vi "Finish.vi"(8 "error in (no error)":errorcluster, 11 "DriverStation in":refnum<class "DriverStation.lvclass">) -> (0 "error out":errorcluster, 3 "DriverStation out":refnum<class "DriverStation.lvclass">)   [LabVIEW 2013, in "DriverStation.lvclass"]
uses:
  DriverStation.lvclass
  System/System.lvclass
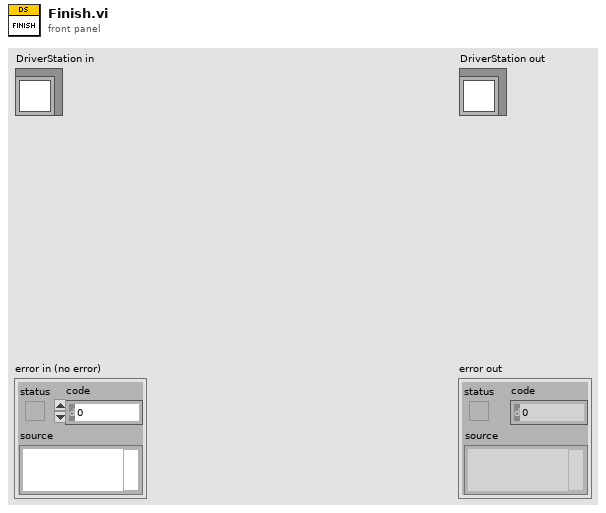
[diagram p1: front panel]
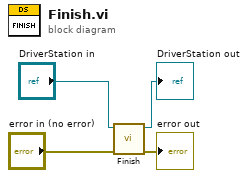
[diagram p0: block diagram]
diagram:
  n1 = call-parent "Finish.vi"("error in (no error)"="error in (no error)", "System in"="DriverStation in") -> ("error out"=→"error out":errorcluster, "System out"=→"DriverStation out":refnum<class "DriverStation.lvclass">)  [unwired: 8 in]
